vi "FindAdjacentSWFolders.vi"() -> (2 "isSVN?":bool[](array[boolean]), 3 "Array":path[](array[path]))   [LabVIEW 2020]
uses:
  Globals/Constants_global.vi
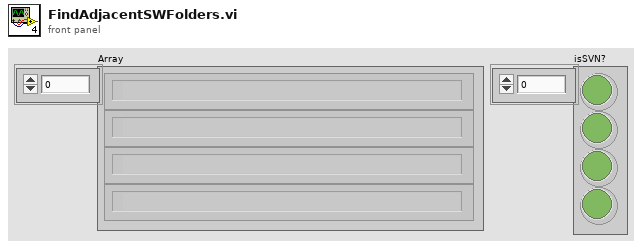
[diagram p1: front panel]
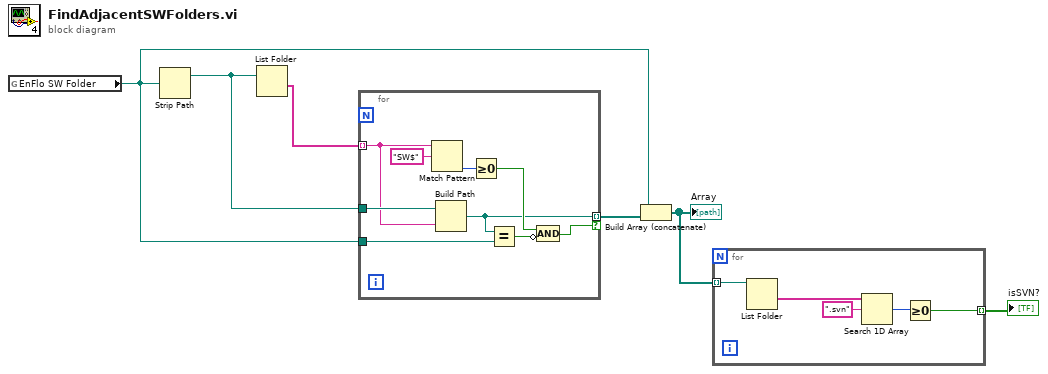
[diagram p0: block diagram]
diagram:
  n1 = global read "Constants_global.vi" "EnFlo SW Folder"() -> (w3:path)
  n2 = Strip Path(path=w3) -> (stripped path=w5:path)  [unwired: 1 out]
  n3 = List Folder(path=w5) -> (folder names=w6:string[])  [unwired: 3 in, 3 out]
  n4 = for {
    tunnel: w6 -> [w13] mode=indexing
    tunnel: w5 -> [w14]
    tunnel: [w10] -> w4 mode=indexing if=w8
    tunnel: w3 -> [w9]
    n5 = Match Pattern(string=w13, regular expression="SW$") -> (offset past match=w12:i32)  [unwired: 1 in, 3 out]
    n6 = Build Path(base path=w14, name or relative path=w13) -> (appended path=w10:path)
    n7 = Greater Or Equal To 0?(x=w12) -> (x >= 0?=w11:bool)
    n8 = Equal?(x=w10, y=w9) -> (x = y?=w7:bool)
    n9 = Compound Arithmetic op=AND(w11, invert w7) -> (w8:bool)
  }
  n10 = Build Array (concatenate)(w3, w4) -> (w2:path[])
  "Array" <- w2
  n11 = for {
    tunnel: w2 -> [w20] mode=indexing
    tunnel: [w16] -> w1 mode=indexing
    n12 = List Folder(path=w20) -> (folder names=w19:string[])  [unwired: 3 in, 3 out]
    n13 = Search 1D Array(1D array=w19, element=".svn") -> (index of element=w17:i32)  [unwired: 1 in]
    n14 = Greater Or Equal To 0?(x=w17) -> (x >= 0?=w16:bool)
  }
  "isSVN?" <- w1
